vi "FPGANic-Tester.vi"() -> ()   [LabVIEW 2017]
uses:
  Source.Machine.Settings.ctl
  FPGANic.Events.ctl
  <vilib>/FPGAPlugInAG/PXIe-6592R/niLvFpga_Open_PXIe-6592R.vi
  <vilib>/rvi/interface/common/dynamic/niFpgaDynamicAddResources.vi
  FPGANic.Globals.vi
  <vilib>/Utility/error.llb/Error Cluster From Error Code.vi
  <vilib>/rvi/errors/niLvFpgaAdjustHostInterfaceError.vi
  <vilib>/FPGAPlugInAG/Dynamic/niLvFpga_Close_Dynamic.vi
  <vilib>/rvi/interface/nirviOpenFPGA/nirviOpenFPGA.xnode
  FPGA Bitfiles/FPGANic-Top.lvbitx
  <vilib>/rvi/interface/nirviMethod/nirviMethod.xnode
  <vilib>/rvi/interface/nirviReadWriteControl/nirviReadWriteControl.xnode
  <vilib>/rvi/interface/nirviCloseFPGA/nirviCloseFPGA.xnode
  <vilib>/FPGAPlugInAG/Dynamic/niLvFpga_ReadFifo_Dynamic.vi
  <vilib>/rvi/errors/niLvFpgaMergeErrorWithErrorCode.vi
  NiFpgaLv.dll
  <vilib>/rvi/interface/Simulation/niFpgaSimulationCallBeginRW.vi
  <vilib>/FPGAPlugInAG/Dynamic/niLvFpga_WriteFifo_Dynamic.vi
panel:
  in  "Read Probes":bool
  in  "Read Debug FIFOs":bool
  in  "Tab Control":T1(tab)
  in  "Ethernet II Params":T2={"Destination MAC"=[0, 2, 201, 85, 8, 68], "Source MAC"=[0, 1, 2, 3, 4, 5], "EtherType"=2048} {"Destination MAC" format="%.0x"; "Source MAC" format="%.02x"; "EtherType" format="%.0x"}
  in  "IPv4 Params":T3={"Destination IP"=[10, 0, 1, 100], "Source IP"=[10, 0, 1, 101], "Protocol"=17}
  in  "UDP Params":T4={"Source Port"=35312, "Destination Port"=35312, "Payload"="ABCD"}
  in  "MAC & IP":T5={"MAC Address"=[0, 1, 2, 3, 4, 5], "IP Address"=[10, 0, 1, 101]} {"MAC Address" format="%.0x"}
  out "Write Probe 2":u64[](array[numeric]) format="%.0x"
  out "Write Probe 1":u64[](array[numeric]) format="%.0x"
  out "Read Probe":u64[](array[numeric]) format="%.0x"
  out "Debug FIFO 2":u32[](array[numeric]) format="%.0x"
  out "Debug FIFO 1":u32[](array[numeric]) format="%.0x"
  out "UDP Payload":u8[](array[numeric]) format="%.0x"
  in  "Clear Debug FIFOS?":bool=TRUE
  in  "AXI_STR_RXD_3_tkeep":u8=15
  out "GPIO #1 out":u32 format="%.0x"
  in  "GPIO #2 in":u32 format="%.0x"
  in  "GPIO #1 in":u32=4 format="%.0x"
  out "GPIO #2 out":u32
  in  "AXI_STR_RXD_3_tkeep":u8=15
  out "sPort0_Power_Good":bool
  out "signal_detect_Port0":bool
  out "aBlockLockPort0":bool
  in  "Read/Write GPIO":bool
  out "error out":errorcluster
  out "Status":string
  in  "error in":errorcluster
  in  "Exit":bool
  in  "Transmit Packet":bool
  in  "Read Packet":bool
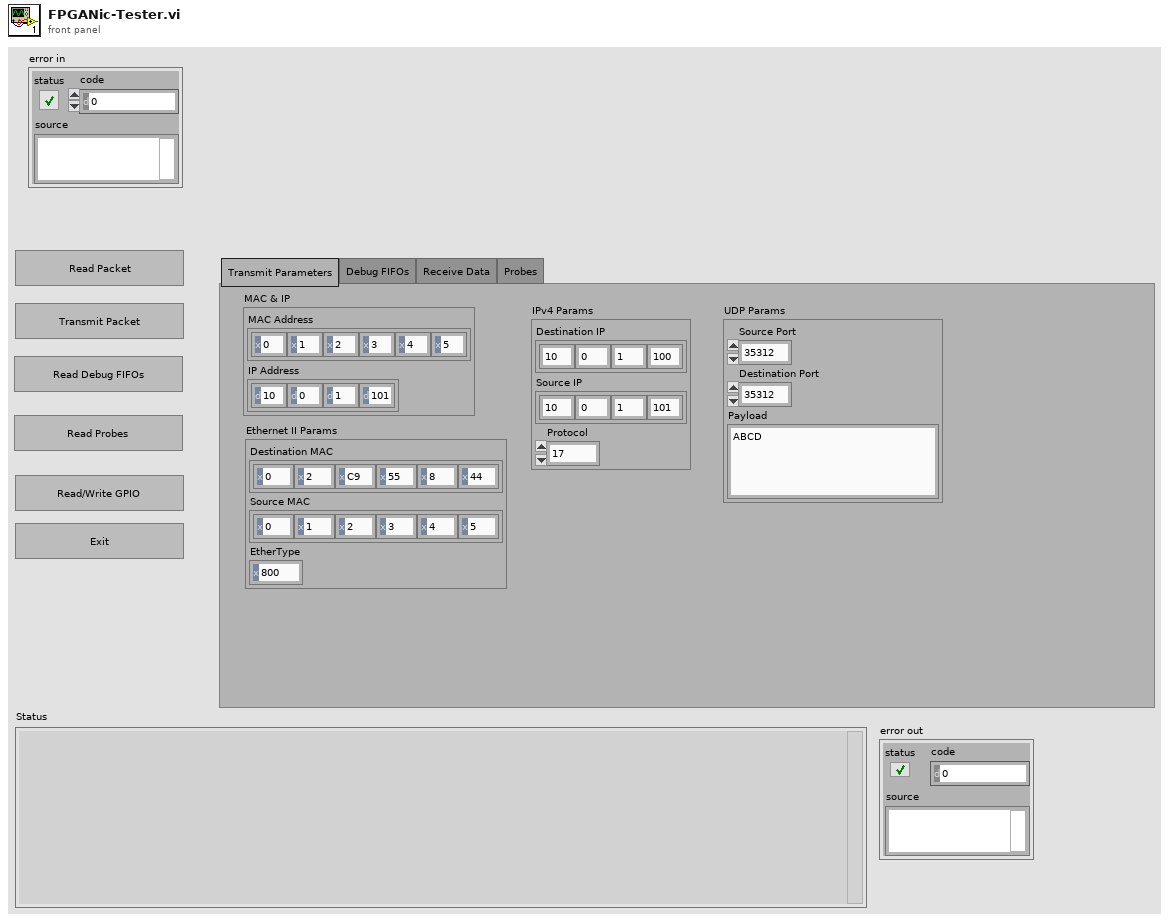
[diagram p1: front panel]
types:
  T1 = enum32{"Transmit Parameters", "Debug FIFOs", "Receive Data", "Probes"}
  T2 = cluster{"Destination MAC":u8[], "Source MAC":u8[], "EtherType":u16}
  T3 = cluster{"Destination IP":u8[], "Source IP":u8[], "Protocol":u8}
  T4 = cluster{"Source Port":u16, "Destination Port":u16, "Payload":string}
  T5 = typedef "Source.Machine.Settings.ctl" = cluster{"MAC Address":u8[], "IP Address":u8[]}
  T6 = typedef "FPGANic.Events.ctl" = enum16{"Open FPGA", "Close FPGA", "Reset UI", "Read Packet", "Transmit Packet", "Read Debug FIFOs", "Read Probes", "Read/Write GPIO"}
  T7 = cluster{"Read Probe":u64[], "Write Probe 1":u64[], "Write Probe 2":u64[], "Debug FIFO 1":u32[], "Debug FIFO 2":u32[]}
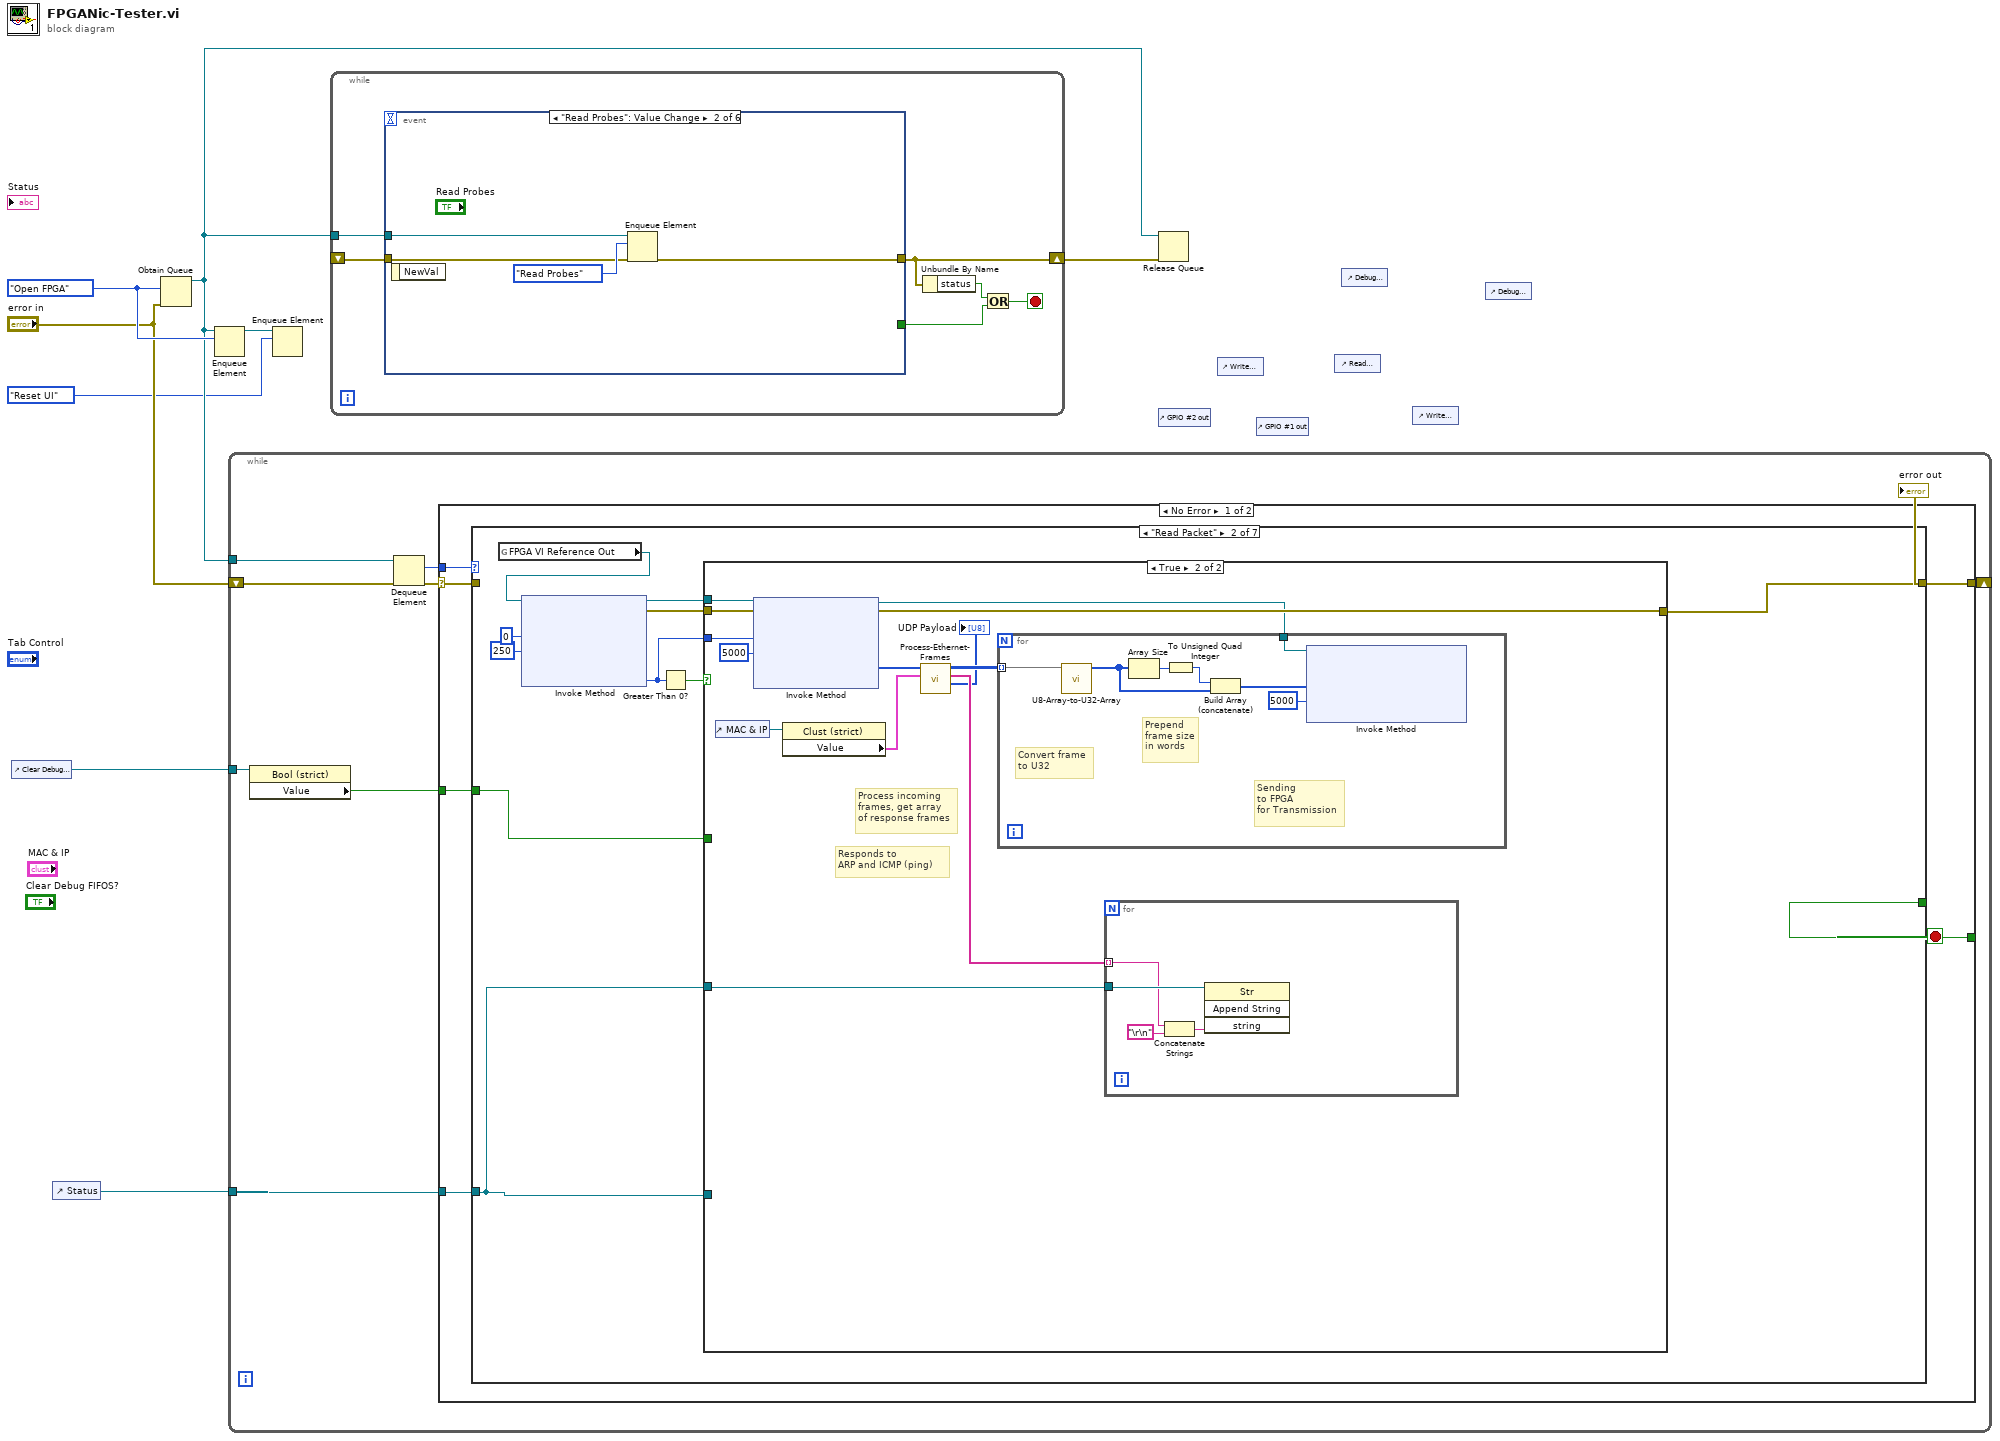
[diagram p0: block diagram]
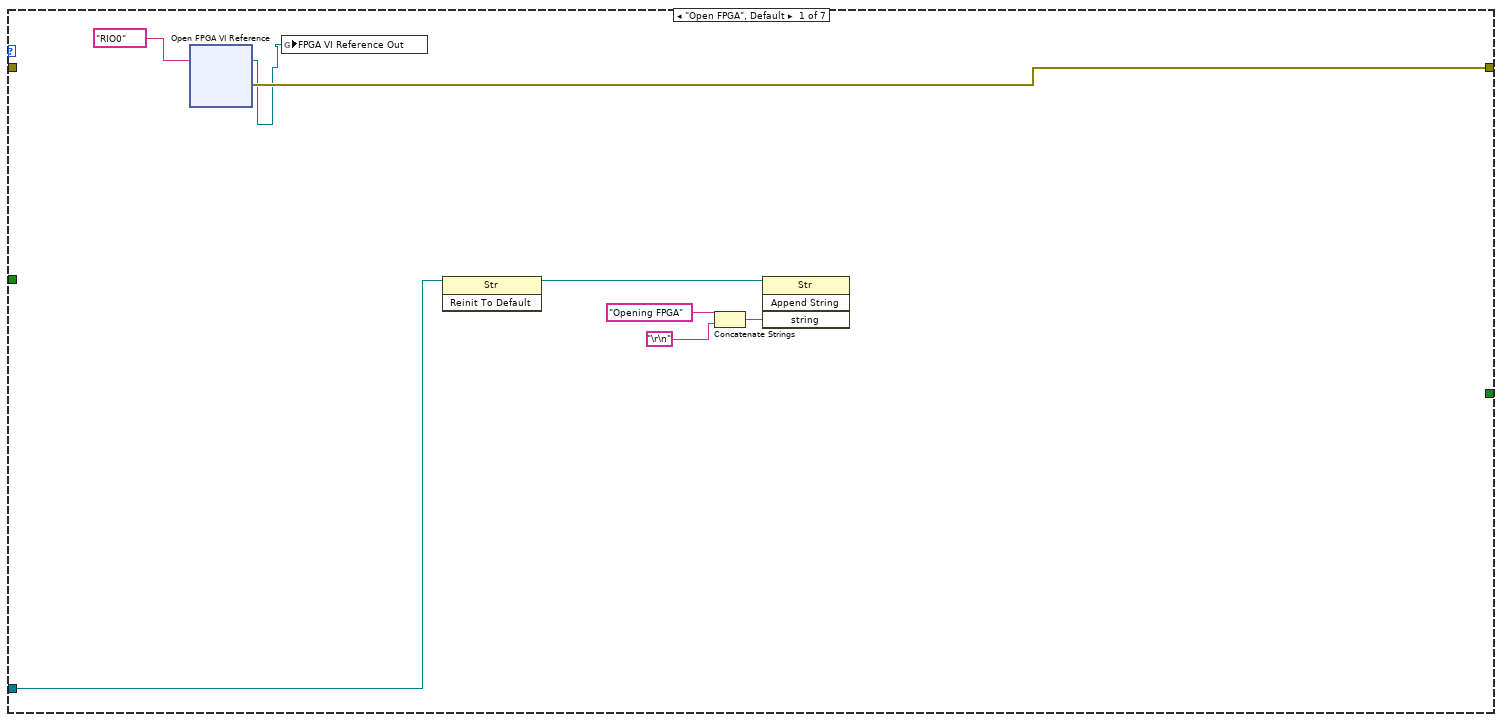
[diagram p2: hidden frame]
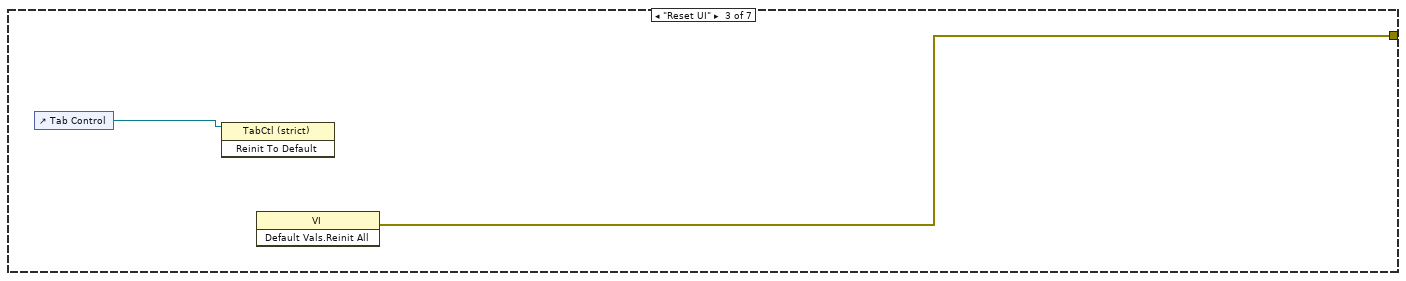
[diagram p4: hidden frame]
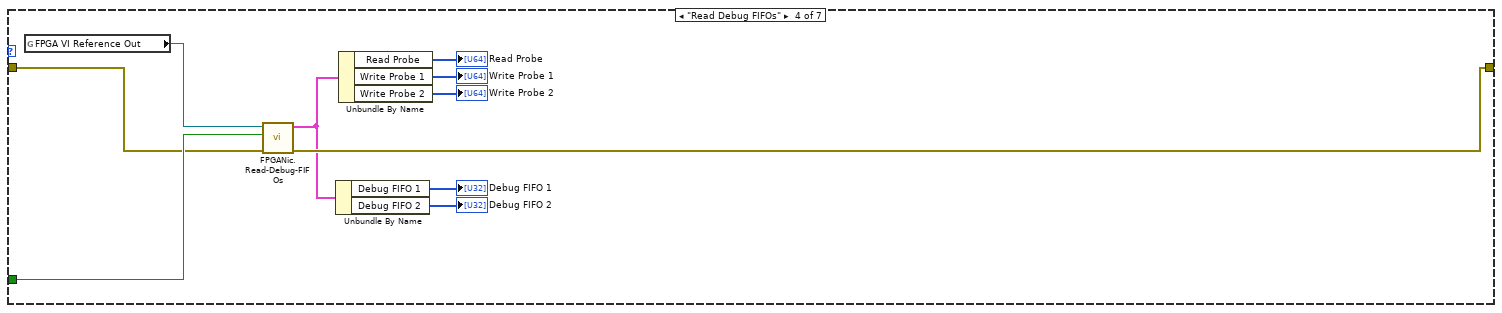
[diagram p5: hidden frame]
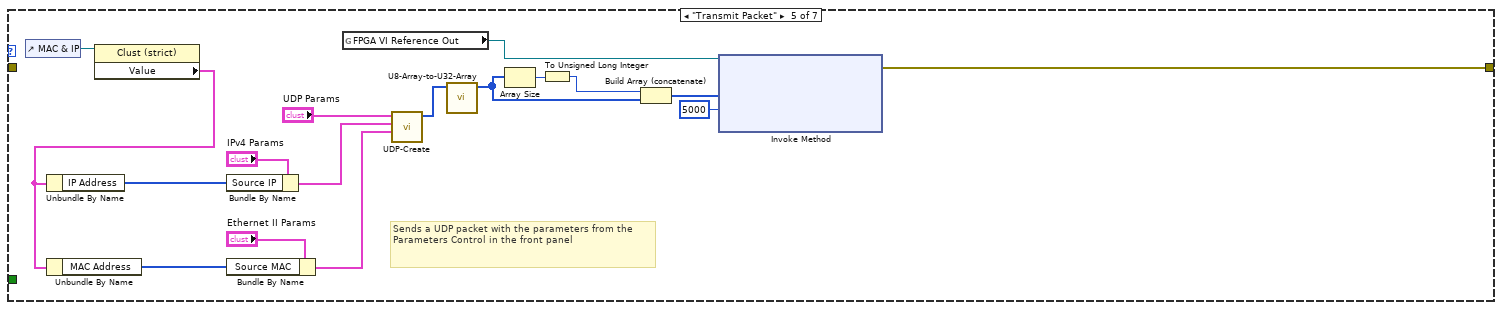
[diagram p6: hidden frame]
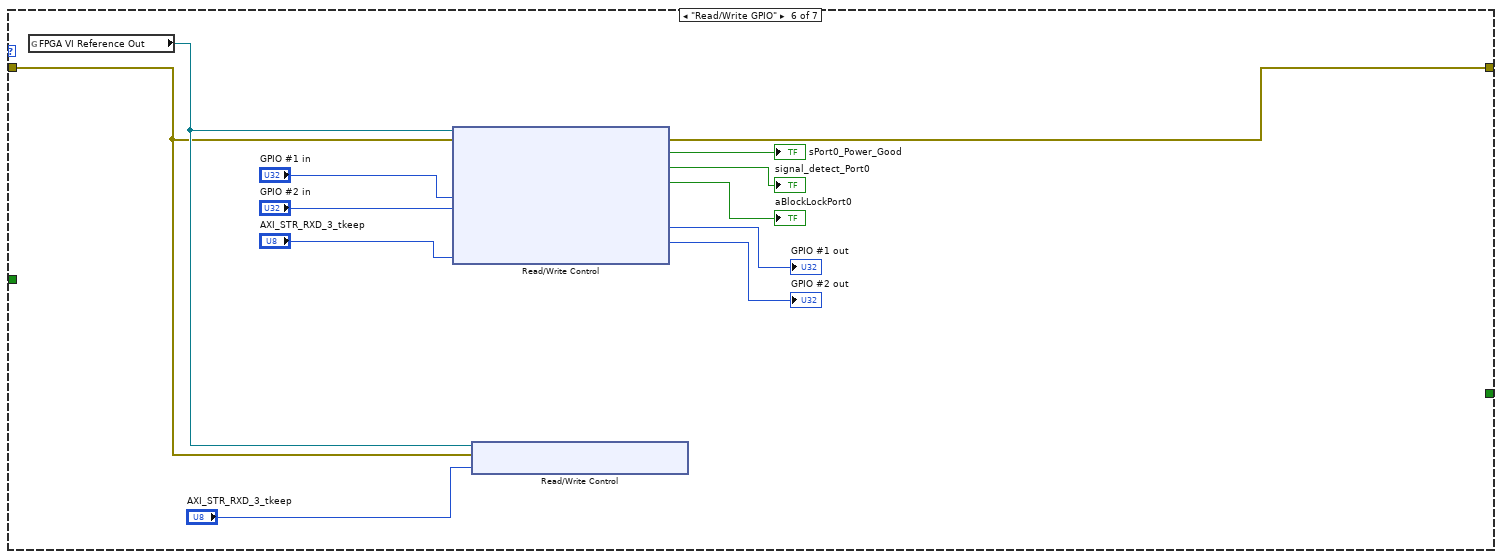
[diagram p7: hidden frame]
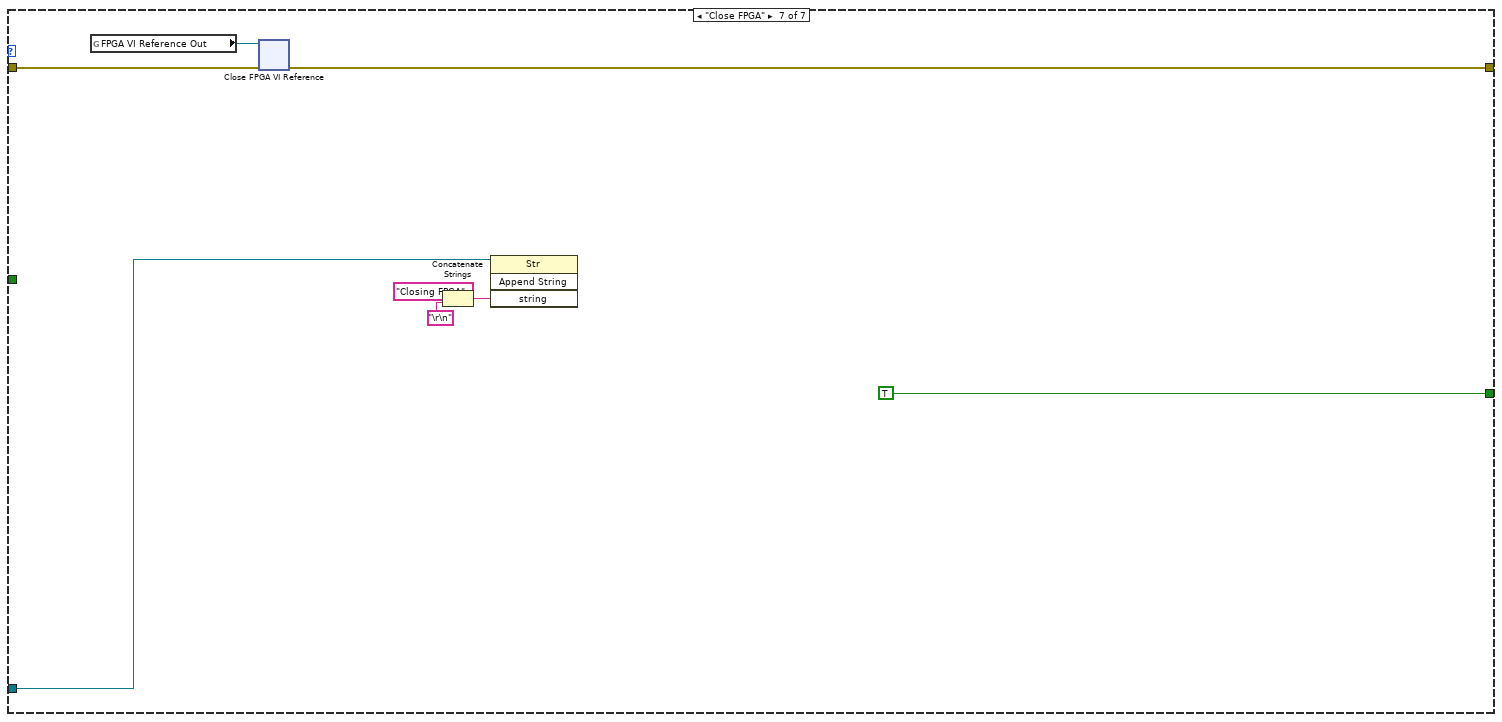
[diagram p8: hidden frame]
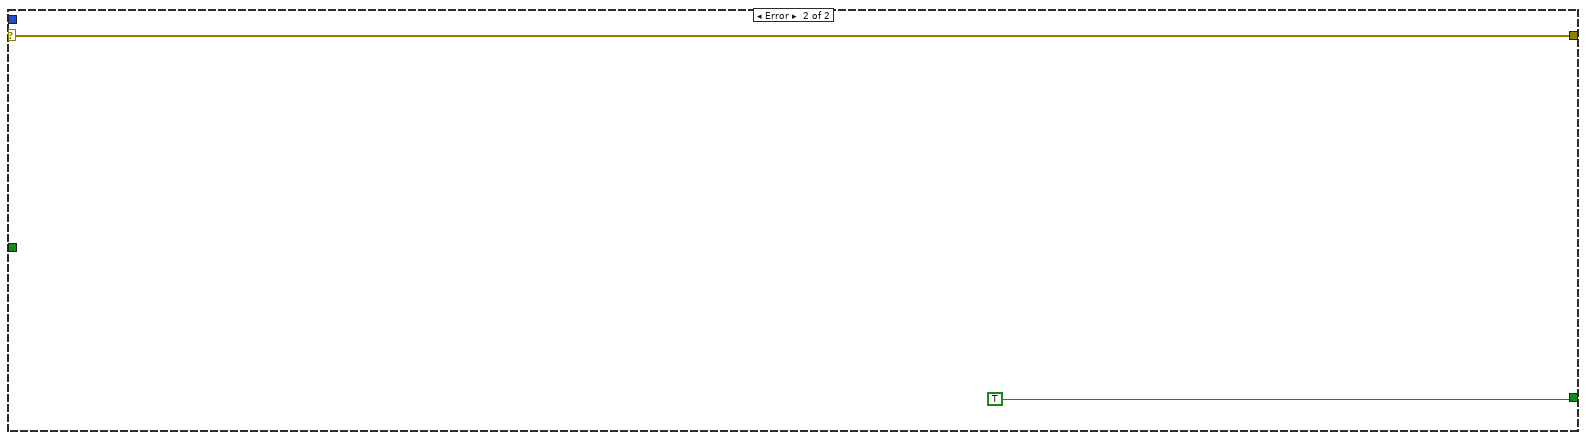
[diagram p9: hidden frame]
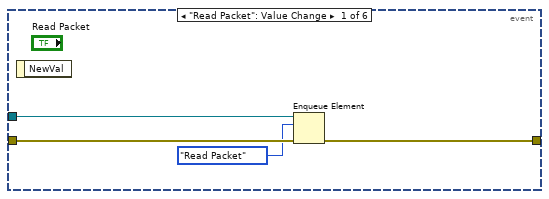
[diagram p10: hidden frame]
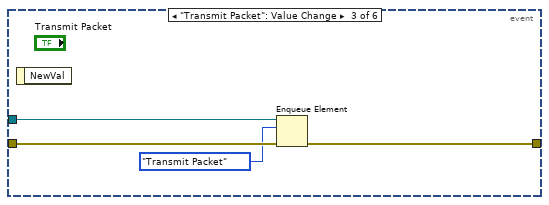
[diagram p11: hidden frame]
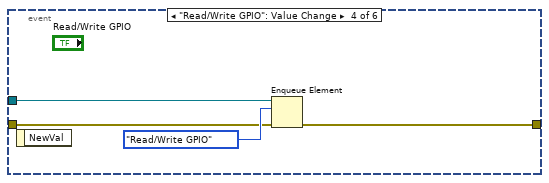
[diagram p12: hidden frame]
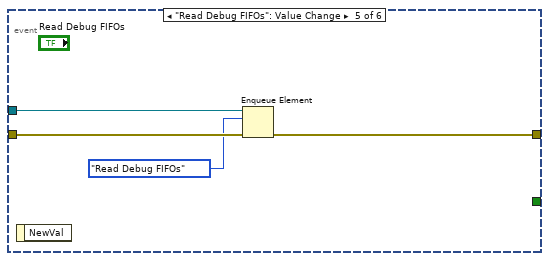
[diagram p13: hidden frame]
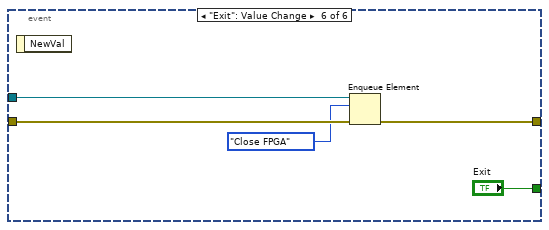
[diagram p14: hidden frame]
diagram:
  w8 = FPGANic.Events."Open FPGA" ("Enum")
  n1 = control-ref of="Clear Debug FIFOS?"() -> (w3:refnum<vi>)
  n2 = control-ref of="Status"() -> (w4:refnum<vi>)
  n3 = Obtain Queue(element data type=w8, error in (no error)="error in") -> (queue out=w6:refnum<queue>)  [unwired: 3 in, 2 out]
  n4 = Enqueue Element(queue=w6, element=w8) -> (queue out=w2:refnum<queue>)  [unwired: 2 in, 2 out]
  n5 = while {
    tunnel: w6 -> [w17]
    shift-right: [w12] -> _
    shift-left: "error in" -> [w13]
    tunnel: w4 -> [w11]
    tunnel: w3 -> [w10]
    stop <- w14 stop-if-true
    n6 = property class="Bool (strict)"(reference=w10) -> ("Value"=w9:bool)  [unwired: 1 in, 2 out]
    n7 = Dequeue Element(queue=w17, error in (no error)=w13) -> (element=w15:T6, error out=w16:errorcluster)  [unwired: 1 in, 2 out]
    n8 = case shown="No Error" w16 {
      selector: w16 -> [w18 w116]
      tunnel: w15 -> [w23 _]
      tunnel: [w22 TRUE] -> w14
      tunnel: [w21 w116] -> w12
      tunnel: w11 -> [w20 _]
      tunnel: w9 -> [w19 _]
      frame No Error {
        n9 = case shown="\"Read Packet\"" w23 {
          tunnel: [_ _ _ _ _ _ TRUE] -> w22
          tunnel: [w31 w36 w67 w76 w93 w99 w114] -> w21
          tunnel: w20 -> [w27 w32 _ _ _ _ w110]
          tunnel: w19 -> [_ w34 _ w77 _ _ _]
          tunnel: w18 -> [_ _ _ w75 _ w96 w108]
          frame "Open FPGA", Default {
            n10 = xnode "Open FPGA VI Reference"("resource name"=tag "RIO0") -> ("FPGA VI Reference Out"=w24:refnum<k20>, "error out"=w31:errorcluster)  [unwired: 1 in]
            n11 = global write "FPGANic.Globals.vi" "FPGA VI Reference Out"(w24) -> ()
            n12 = invoke class="Str" method="Reinit To Default"(reference=w27) -> (reference out=w26:refnum<vi>)  [unwired: 2 in, 2 out]
            n13 = Concatenate Strings("Opening FPGA" ("string"), "\r\n") -> (w30:string)
            n14 = invoke class="Str" method="Append String"(reference=w26, "string"=w30) -> ()  [unwired: 2 in, 4 out]
          }
          frame "Read Packet" {
            n15 = global read "FPGANic.Globals.vi" "FPGA VI Reference Out"() -> (w33:refnum<k20>)
            n16 = xnode "Invoke Method"("FPGA VI Reference In"=w33, "Number of Elements"=u32 0, "Timeout (ms)"=250) -> ("FPGA VI Reference Out"=w38:refnum<k20>, "error out"=w37:errorcluster, "Elements Remaining"=w35:u32)  [unwired: 1 in, 1 out]
            n17 = Greater Than 0?(x=w35) -> (x > 0?=w39:bool)
            n18 = case shown="True" w39 {
              tunnel: w38 -> [_ w54]
              tunnel: w37 -> [w42 w53]
              tunnel: [w42 w51] -> w36
              tunnel: w32 -> [_ _]
              tunnel: w35 -> [_ w52]
              tunnel: w34 -> [_ _]
              tunnel: w32 -> [_ w45]
              frame False {
              }
              frame True {
                # "Responds to\nARP and ICMP (ping)"
                # "Process incoming\nframes, get array\nof response frames"
                n19 = control-ref of="MAC & IP"() -> (w48:refnum<vi>)
                n20 = xnode "Invoke Method"("FPGA VI Reference In"=w54, "error in"=w53, "Number of Elements"=w52, "Timeout (ms)"=5000) -> ("FPGA VI Reference Out"=w46:refnum<k20>, "error out"=w51:errorcluster, "Data"=w50:u64[])  [unwired: 1 out]
                n21 = property class="Clust (strict)"(reference=w48) -> ("Value"=w47:T5)  [unwired: 1 in, 2 out]
                n22 = call "Process-Ethernet-Frames.vi"("Source Machine\nSettings"=w47, "Raw Data\nStream"=w50) -> ("UDP Payload"=→"UDP Payload":u8[], "Messages"=w44:string[], "Frames to send"=w49:u8[][])  [unwired: 7 in]
                n23 = for {
                  tunnel: w49 -> [w66] mode=indexing
                  tunnel: w46 -> [w60]
                  # "Prepend\nframe size\nin words"
                  # "Sending\nto FPGA\nfor Transmission"
                  # "Convert frame\nto U32"
                  n24 = call "U8-Array-to-U32-Array.vi"("Frame U8[] in"=w66) -> ("Frame U32[] out"=w61:u32[])  [unwired: 10 in]
                  n25 = Array Size(array=w61) -> (size(s)=w65:i32)
                  n26 = To Unsigned Quad Integer(1:w65) -> (0:w64:u64)
                  n27 = Build Array (concatenate)(w64, w61) -> (w63:u64[])
                  n28 = xnode "Invoke Method"("FPGA VI Reference In"=w60, "Data"=w63, "Timeout (ms)"=5000) -> ()  [unwired: 1 in, 3 out]
                }
                n29 = for {
                  tunnel: w45 -> [w57]
                  tunnel: w44 -> [w56] mode=indexing
                  n30 = Concatenate Strings(w56, "\r\n") -> (w59:string)
                  n31 = invoke class="Str" method="Append String"(reference=w57, "string"=w59) -> ()  [unwired: 2 in, 4 out]
                }
              }
            }
          }
          frame "Reset UI" {
            n32 = control-ref of="Tab Control"() -> (w68:refnum<vi>)
            n33 = invoke class="TabCtl (strict)" method="Reinit To Default"(reference=w68) -> ()  [unwired: 2 in, 3 out]
            n34 = invoke class="VI" method="Default Vals.Reinit All"() -> (error out=w67:errorcluster)  [unwired: 3 in, 2 out]
          }
          frame "Read Debug FIFOs" {
            n35 = global read "FPGANic.Globals.vi" "FPGA VI Reference Out"() -> (w78:refnum<k20>)
            n36 = call "FPGANic.Read-Debug-FIFOs.vi"("error in"=w75, "Value"=w77, "Refnum in"=w78) -> ("error out"=w76:errorcluster, "Debug Data"=w71:T7)  [unwired: 7 in]
            n37 = Unbundle By Name(w71) -> ("Debug FIFO 1"=→"Debug FIFO 1":u32[], "Debug FIFO 2"=→"Debug FIFO 2":u32[])
            n38 = Unbundle By Name(w71) -> ("Read Probe"=→"Read Probe":u64[], "Write Probe 1"=→"Write Probe 1":u64[], "Write Probe 2"=→"Write Probe 2":u64[])
          }
          frame "Transmit Packet" {
            # "Sends a UDP packet with the parameters from the\nParameters Control in the front panel"
            n39 = control-ref of="MAC & IP"() -> (w82:refnum<vi>)
            n40 = property class="Clust (strict)"(reference=w82) -> ("Value"=w80:T5)  [unwired: 1 in, 2 out]
            n41 = Unbundle By Name(w80) -> ("IP Address"=w81:u8[])
            n42 = Unbundle By Name(w80) -> ("MAC Address"=w79:u8[])
            n43 = Bundle By Name(cluster="IPv4 Params", "Source IP"=w81) -> (w83:T3)
            n44 = Bundle By Name(cluster="Ethernet II Params", "Source MAC"=w79) -> (w84:T2)
            n45 = global read "FPGANic.Globals.vi" "FPGA VI Reference Out"() -> (w92:refnum<k20>)
            n46 = call "UDP-Create.vi"("Ethernet II Params"=w84, "IPv4 Params"=w83, "UDP Params"="UDP Params") -> ("Ethernet Frame"=w91:u8[])  [unwired: 6 in, 2 out]
            n47 = call "U8-Array-to-U32-Array.vi"("Frame U8[] in"=w91) -> ("Frame U32[] out"=w88:u32[])  [unwired: 10 in]
            n48 = Array Size(array=w88) -> (size(s)=w90:i32)
            n49 = To Unsigned Long Integer(number=w90) -> (unsigned 32bit integer=w89:u32)
            n50 = Build Array (concatenate)(w89, w88) -> (w87:u32[])
            n51 = xnode "Invoke Method"("FPGA VI Reference In"=w92, "Data"=w87, "Timeout (ms)"=5000) -> ("error out"=w93:errorcluster)  [unwired: 1 in, 2 out]
          }
          frame "Read/Write GPIO" {
            n52 = global read "FPGANic.Globals.vi" "FPGA VI Reference Out"() -> (w97:refnum<k20>)
            n53 = xnode "Read/Write Control"("FPGA VI Reference In"=w97, "error in"=w96, "GPIO #1 in"="GPIO #1 in", "GPIO #2 in"="GPIO #2 in", "d_microblaze_i\\AXI_STR_RXD_3_tkeep"="AXI_STR_RXD_3_tkeep") -> ("error out"=w99:errorcluster, "sPort0_Power_Good"=→"sPort0_Power_Good":bool, "signal_detect_Port0"=→"signal_detect_Port0":bool, "aBlockLockPort0"=→"aBlockLockPort0":bool, "GPIO #1 out"=→"GPIO #1 out":u32, "GPIO #2 out"=→"GPIO #2 out":u32)  [unwired: 1 out]
            n54 = xnode "Read/Write Control"("FPGA VI Reference In"=w97, "error in"=w96, "d_microblaze_i\\AXI_STR_RXD_3_tkeep"="AXI_STR_RXD_3_tkeep") -> ()  [unwired: 2 out]
          }
          frame "Close FPGA" {
            n55 = global read "FPGANic.Globals.vi" "FPGA VI Reference Out"() -> (w109:refnum<k20>)
            n56 = xnode "Close FPGA VI Reference"("FPGA VI Reference In"=w109, "error in"=w108) -> ("error out"=w114:errorcluster)
            n57 = Concatenate Strings("Closing FPGA" ("string"), "\r\n") -> (w113:string)
            n58 = invoke class="Str" method="Append String"(reference=w110, "string"=w113) -> ()  [unwired: 2 in, 4 out]
          }
        }
      }
      frame Error {
      }
    }
    "error out" <- w12
  }
  n59 = Enqueue Element(queue=w2, element=FPGANic.Events."Reset UI" ("Enum")) -> ()  [unwired: 2 in, 3 out]
  n60 = while {
    tunnel: w6 -> [w123]
    shift-right: [w118] -> w7
    shift-left: _ -> [w119]
    stop <- w121 stop-if-true
    n61 = event shown="[1] \"Read Probes\": Value Change" {
      selector: _ -> [_ _ _ _ _ _]
      dyn-events: _ -> [_ _ _ _ _ _]
      timeout: _ -> [_ _ _ _ _ _]
      tunnel: w123 -> [w127 w128 w135 w138 w143 w148]
      tunnel: [w126 w129 w133 w136 w140 w147] -> w118
      tunnel: [_ _ _ _ _ "Exit"] -> w120
      tunnel: w119 -> [w125 w130 w134 w137 w142 w145]
      event "Read Packet": Value Change {
        n62 = event-data() -> ()  [unwired: 1 in, 1 out]
        n63 = Enqueue Element(queue=w127, element=FPGANic.Events."Read Packet" ("Enum"), error in (no error)=w125) -> (error out=w126:errorcluster)  [unwired: 1 in, 2 out]
      }
      event "Read Probes": Value Change {
        n64 = event-data() -> ()  [unwired: 1 in, 1 out]
        n65 = Enqueue Element(queue=w128, element=FPGANic.Events."Read Probes" ("Enum"), error in (no error)=w130) -> (error out=w129:errorcluster)  [unwired: 1 in, 2 out]
      }
      event "Transmit Packet": Value Change {
        n66 = event-data() -> ()  [unwired: 1 in, 1 out]
        n67 = Enqueue Element(queue=w135, element=FPGANic.Events."Transmit Packet" ("Enum"), error in (no error)=w134) -> (error out=w133:errorcluster)  [unwired: 1 in, 2 out]
      }
      event "Read/Write GPIO": Value Change {
        n68 = event-data() -> ()  [unwired: 1 in, 1 out]
        n69 = Enqueue Element(queue=w138, element=FPGANic.Events."Read/Write GPIO" ("Enum"), error in (no error)=w137) -> (error out=w136:errorcluster)  [unwired: 1 in, 2 out]
      }
      event "Read Debug FIFOs": Value Change {
        n70 = event-data() -> ()  [unwired: 1 in, 1 out]
        n71 = Enqueue Element(queue=w143, element=FPGANic.Events."Read Debug FIFOs" ("Enum"), error in (no error)=w142) -> (error out=w140:errorcluster)  [unwired: 1 in, 2 out]
      }
      event "Exit": Value Change {
        n72 = event-data() -> ()  [unwired: 1 in, 1 out]
        n73 = Enqueue Element(queue=w148, element=FPGANic.Events."Close FPGA" ("Enum"), error in (no error)=w145) -> (error out=w147:errorcluster)  [unwired: 1 in, 2 out]
      }
    }
    n74 = Unbundle By Name(w118) -> ("status"=w122:bool)
    n75 = Or(x=w122, y=w120) -> (x .or. y?=w121:bool)
  }
  n76 = Release Queue(queue=w6, error in (no error)=w7) -> ()  [unwired: 1 in, 3 out]
  n77 = control-ref of="GPIO #2 out"() -> ()  [unwired: 1 out]
  n78 = control-ref of="Write Probe 1"() -> ()  [unwired: 1 out]
  n79 = control-ref of="GPIO #1 out"() -> ()  [unwired: 1 out]
  n80 = control-ref of="Read Probe"() -> ()  [unwired: 1 out]
  n81 = control-ref of="Debug FIFO 1"() -> ()  [unwired: 1 out]
  n82 = control-ref of="Write Probe 2"() -> ()  [unwired: 1 out]
  n83 = control-ref of="Debug FIFO 2"() -> ()  [unwired: 1 out]
